vi "macro_BangBang_Execute.vi"   [LabVIEW 2019, in "Trajectory_Library.lvlib"]
uses:
  Trajectory_Library.lvlib
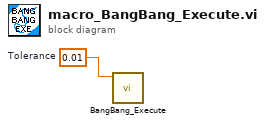
[diagram p0: block diagram]
diagram:
  w1 = 0.01  # Tolerance
  n1 = call "BangBang_Execute.vi"("Tolerance"=w1) -> ()  [unwired: 8 in, 3 out]
